vi "Format Data.vi"(6 "Raw?":bool, 7 "Inidicies":i32[](array[numeric]), 8 "Reset":bool, 9 "data":waveform(dbl)[](array[waveform]), 10 "T_0 Index":i32, 11 "Active Channels":string[][](array[string])) -> (0 "AI Chan Avg.":string[](array[string]), 1 "Temperature Avg":dbl[](array[numeric]), 2 "Temperatre Plot Data":cluster{dbl[], i32[]}[](array[cluster]), 3 "Data Out":waveform(dbl)[](array[waveform]), 4 "data ready":bool, 5 "Torque":dbl)   [LabVIEW 2017]
uses:
  <vilib>/Analysis/baseanly.llb/Mean (DBL).vi
  <vilib>/Analysis/NI_AALBase.lvlib
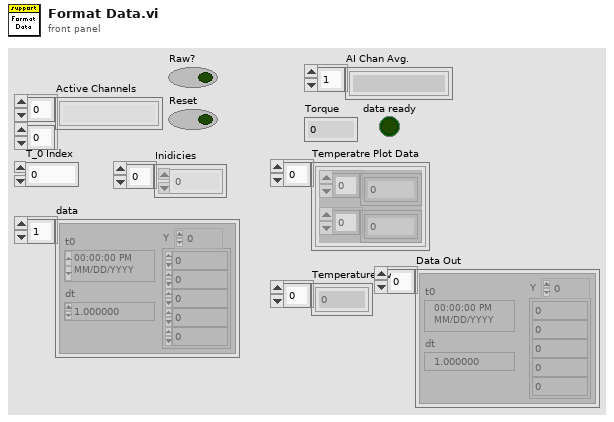
[diagram p1: front panel]
types:
  T1 = cluster{"window for DC":enum16{"Rectangular (none)", "Hanning", "Low side lobe"}, "output function":enum16{"DC only", "RMS only", "DC and RMS"}, "window for RMS":enum16{"Rectangular (none)", "Hanning", "Low side lobe"}, "exp. time constant":dbl, "Ignore input start time":bool}
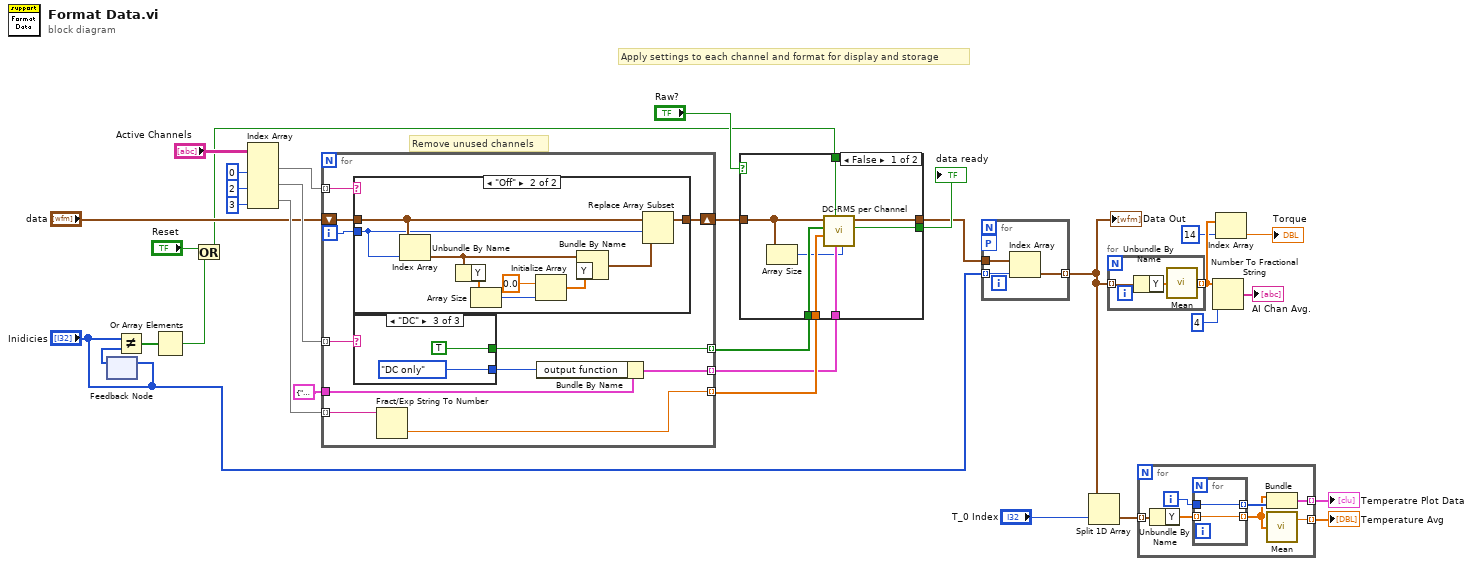
[diagram p0: block diagram]
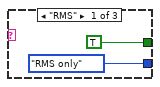
[diagram p3: hidden frame]
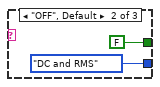
[diagram p4: hidden frame]
diagram:
  # "Remove unused channels"
  # "Apply settings to each channel and format for display and storage"
  n1 = feedback-in #1("Inidicies") -> ()
  n2 = feedback #1() -> (w22:i32[])  [unwired: 1 in]
  n3 = Not Equal?(x="Inidicies", y=w22) -> (x != y?=w21:bool[])
  n4 = Or Array Elements(Boolean array=w21) -> (logical OR=w20:bool)
  n5 = Or(x="Reset", y=w20) -> (x .or. y?=w5:bool)
  n6 = Index Array(array="Active Channels", index (col) #1=0 ("disabled index (col)"), index (col) #2=2 ("disabled index (col)"), index (col) #3=3 ("index (col)")) -> (element #1=w16:string[], element #2=w15:string[], element #3=w14:string[])  [unwired: 3 in]
  n7 = for {
    shift-right: [w42] -> w9
    shift-left: "data" -> [w43]
    tunnel: w16 -> [w41] mode=indexing
    tunnel: w15 -> [w39] mode=indexing
    tunnel: w14 -> [w38] mode=indexing
    tunnel: T1 {"window for DC"=enum."Rectangular (none)", "output function"=enum."DC and RMS", "window for RMS"=enum."Rectangular (none)", "exp. time constant"=-1.0, "Ignore input start time"=FALSE} ("averaging control") -> [w37]
    tunnel: [w35] -> w12 mode=indexing
    tunnel: [w34] -> w10 mode=indexing
    tunnel: [w33] -> w11 mode=indexing
    i -> [w40]
    n8 = case shown="\"Off\"" w41 {
      tunnel: w43 -> [w50 w54]
      tunnel: [w50 w53] -> w42
      tunnel: w40 -> [_ w51]
      frame Default {
      }
      frame "Off" {
        n9 = Index Array(array=w54, index=w51) -> (element=w59:waveform(dbl))
        n10 = Unbundle By Name(w59) -> ("Y"=w58:dbl[])
        n11 = Array Size(array=w58) -> (size(s)=w56:i32)
        n12 = Initialize Array(0.0, w56) -> (w57:dbl[])
        n13 = Bundle By Name(cluster=w59, "Y"=w57) -> (w52:waveform(dbl))
        n14 = Replace Array Subset(array=w54, new element=w52, index=w51) -> (w53:waveform(dbl)[])
      }
    }
    n15 = case shown="\"DC\"" w39 {
      tunnel: [enum16{"DC only", "RMS only", "DC and RMS"}."RMS only" ("output function") enum16{"DC only", "RMS only", "DC and RMS"}."DC and RMS" ("output function") enum16{"DC only", "RMS only", "DC and RMS"}."DC only" ("output function")] -> w36
      tunnel: [TRUE FALSE TRUE] -> w35
      frame "RMS" {
      }
      frame "OFF", Default {
      }
      frame "DC" {
      }
    }
    n16 = Fract/Exp String To Number(string=w38) -> (number=w33:dbl)  [unwired: 3 in, 1 out]
    n17 = Bundle By Name(cluster=w37, "output function"=w36) -> (w34:T1)
  }
  n18 = case shown="False" "Raw?" {
    selector: "Raw?" -> [_ w68]
    tunnel: [w67 w69] -> w2
    tunnel: w5 -> [w66 _]
    tunnel: w12 -> [w65 _]
    tunnel: w11 -> [w64 _]
    tunnel: w10 -> [w63 _]
    tunnel: w9 -> [w62 w69]
    tunnel: [w60 w68] -> w6
    frame False {
      n19 = Array Size(array=w62) -> (size(s)=w61:i32)
      n20 = call "DC-RMS per Channel.vi"("Array Length"=w61, "Measurement Control"=w63, "reset"=w66, "Averaging Time"=w64, "Enable"=w65, "signals in"=w62) -> ("data ready"=w60:bool, "DC value waveforms"=w67:waveform(dbl)[])  [unwired: 3 in, 1 out]
    }
    frame True {
    }
  }
  "data ready" <- w6
  n21 = for {
    tunnel: w2 -> [w72]
    tunnel: "Inidicies" -> [w71] mode=indexing
    tunnel: [w70] -> w1 mode=indexing
    workers-P: _ -> [_]
    n22 = Index Array(array=w72, index=w71) -> (element=w70:waveform(dbl))
  }
  "Data Out" <- w1
  n23 = Split 1D Array(array=w1, index="T_0 Index") -> (second subarray=w29:waveform(dbl)[])  [unwired: 1 out]
  n24 = for {
    tunnel: w1 -> [w75] mode=indexing
    tunnel: [w73] -> w25 mode=indexing
    n25 = Unbundle By Name(w75) -> ("Y"=w74:dbl[])
    n26 = call-poly <vilib>:"Mean.vi"("X"=w74) -> ("mean"=w73:dbl)  [unwired: 1 out]
  }
  n27 = for {
    tunnel: w29 -> [w82] mode=indexing
    tunnel: [w80] -> w31 mode=indexing
    tunnel: [w76] -> w30 mode=indexing
    i -> [w79]
    n28 = Unbundle By Name(w82) -> ("Y"=w81:dbl[])
    n29 = for {
      tunnel: [w84] -> w77 mode=indexing
      tunnel: w81 -> [w84] mode=indexing
      tunnel: [w83] -> w78 mode=indexing
      tunnel: w79 -> [w83]
    }
    n30 = Bundle(w77, w78) -> (w80:cluster{dbl[], i32[]})  [unwired: 1 in]
    n31 = call-poly <vilib>:"Mean.vi"("X"=w77) -> ("mean"=w76:dbl)  [unwired: 1 out]
  }
  "Temperatre Plot Data" <- w31
  "Temperature Avg" <- w30
  n32 = Number To Fractional String(number=w25, precision (6)=i16 4) -> (F-format string=→"AI Chan Avg.":string[])  [unwired: 2 in]
  n33 = Index Array(array=w25, index=14) -> (element=→"Torque":dbl)
